vi "Get max string length.vi"(8 "error in (no error)":errorcluster, 10 "Font (13pt App)":T1={"Font Name"="App Font", "Size"=13, "Bold"=FALSE, "Italic"=FALSE, "Underline"=FALSE, "Strikeout"=FALSE, "Color"=0}, 11 "Array of strings":string[](array[string])) -> (0 "error out":errorcluster, 3 "max width (pixels)":u32)   [LabVIEW 2012, in "ListBox_XControl.xctl"]
doc: "Uses a free label with autosizing enabled to determine the pixel size of a string using text value and font."
uses:
  ListBox_XControl.xctl
  <vilib>/Utility/miscctls.llb/LVFontTypeDef.ctl
panel:
  # "This free label is used for sizing:\n(Autosizing must me enabled)"
  # "Default"
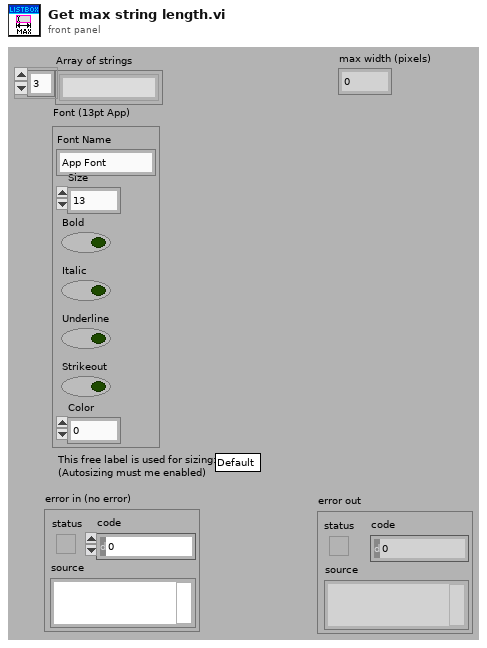
[diagram p1: front panel]
types:
  T1 = typedef "LVFontTypeDef.ctl" = cluster{"Font Name":string, "Size":u16, "Bold":bool, "Italic":bool, "Underline":bool, "Strikeout":bool, "Color":u32}
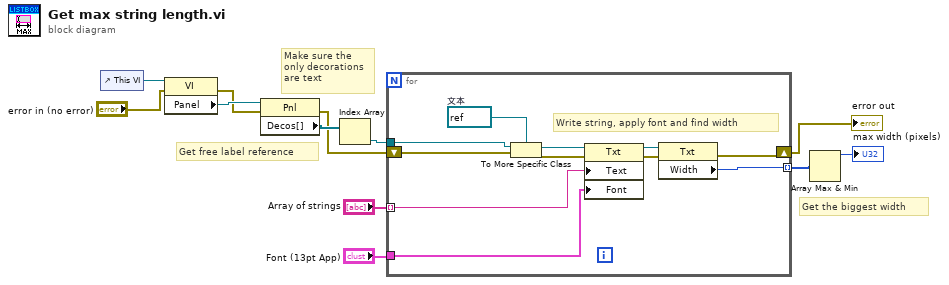
[diagram p0: block diagram]
diagram:
  # "Make sure the only decorations are text"
  # "Get the biggest width"
  # "Get free label reference"
  n1 = control-ref of="This VI"() -> (w12:refnum<vi>)
  n2 = property class="VI"(reference=w12, error in="error in (no error)") -> (error out=w10:errorcluster, "Panel"=w11:refnum<vi>)  [unwired: 1 out]
  n3 = property class="Pnl"(reference=w11, error in=w10) -> (error out=w4:errorcluster, "Decos[]"=w8:refnum<vi>[])  [unwired: 1 out]
  n4 = Index Array(array=w8) -> (element=w7:refnum<vi>)  [unwired: 1 in]
  n5 = for {
    tunnel: w7 -> [w13]
    shift-right: [w18] -> w2
    shift-left: w4 -> [w14]
    tunnel: "Font (13pt App)" -> [w15]
    tunnel: [w17] -> w9 mode=indexing
    tunnel: "Array of strings" -> [w16] mode=indexing
    w23 = refnum<vi> refnum  # 文本
    # "Write string, apply font and find width"
    n6 = To More Specific Class(target class=w23, reference=w13, error in=w14) -> (specific class reference=w22:refnum<vi>, error out=w21:errorcluster)
    n7 = property class="Txt"(reference=w22, error in=w21, "Text"=w16, "Font"=w15) -> (reference out=w20:refnum<vi>, error out=w19:errorcluster)
    n8 = property class="Txt"(reference=w20, error in=w19) -> (error out=w18:errorcluster, "Width"=w17:u32)  [unwired: 1 out]
  }
  "error out" <- w2
  n9 = Array Max & Min(array=w9) -> (max value=→"max width (pixels)":u32)  [unwired: 3 out]
